vi "set_binding_paths.vi"(8 "error in (no error)":errorcluster, 9 "OME header import string ref":refnum<k21>, 10 "notebook import string ref":refnum<k21>, 11 "DataCollectionDL091104Scaffold in":refnum<class "DataCollectionDL091104Scaffold.lvclass">) -> (0 "error out":errorcluster, 3 "DataCollectionDL091104Scaffold out":refnum<class "DataCollectionDL091104Scaffold.lvclass">)   [LabVIEW 2010, in "DataCollectionDL091104Scaffold.lvclass"]
doc: "This method sets the data-binding paths (for the Shared Variable Enginge) for the import strings for the OME header and the notebook. By binding the two import strings to shared variables populated by software on some other computer, additional information for the file header or the notebook can be imported."
uses:
  DataCollectionDL091104Scaffold.lvclass
  DataCollectionDL091104Scaffold.lvclass/DataCollectionDL091104Scaffold.ctl
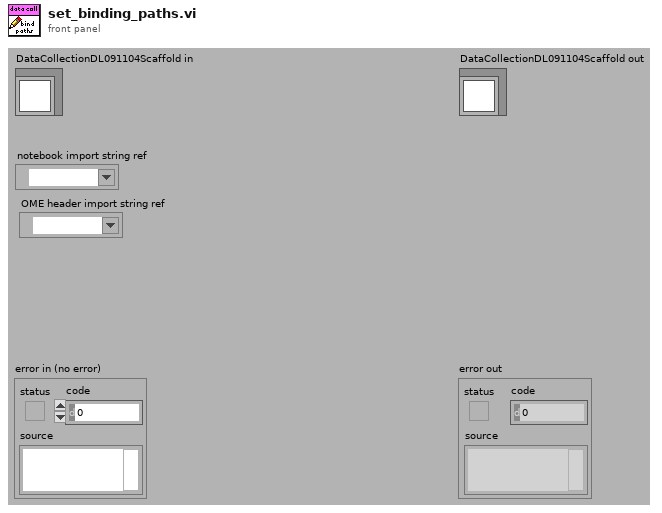
[diagram p1: front panel]
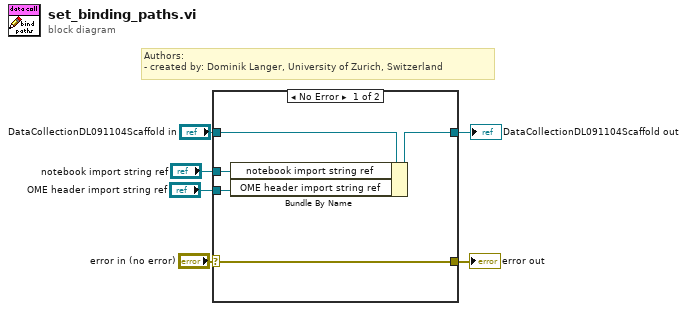
[diagram p0: block diagram]
diagram:
  # "Authors: \n- created by: Dominik Langer, University of Zurich, Switzerland"
  n1 = case shown="No Error" "error in (no error)" {
    selector: "error in (no error)" -> [w8 w13]
    tunnel: [w8 w13] -> w5
    tunnel: [w9 w12] -> w3
    tunnel: "DataCollectionDL091104Scaffold in" -> [w10 w12]
    tunnel: "notebook import string ref" -> [w11 _]
    tunnel: "OME header import string ref" -> [w7 _]
    frame No Error {
      n2 = Bundle By Name(cluster=w10, "notebook import string ref"=w11, "OME header import string ref"=w7) -> (w9:refnum<class "DataCollectionDL091104Scaffold.lvclass">)
    }
    frame Error {
    }
  }
  "error out" <- w5
  "DataCollectionDL091104Scaffold out" <- w3
